vi "Get Next.vi"(0 "Stop Loop in":refnum<class "Stop Loop.lvclass">, 1 "Linked List Ref":refnum<data-value>, 5 "Active Unique ID":string, 9 "Active Element Index":i32, 11 "error in (no error)":errorcluster) -> (3 "Linked List Ref out":refnum<data-value>, 4 "Executioner out":refnum<class "Executioner.lvclass">, 6 "Active Unique ID out":string, 8 "Test Executive Ref out":refnum<data-value>, 10 "Active Element Index out":i32, 12 "Found":bool, 13 "Complete":bool, 14 "Stop":bool, 15 "error out":errorcluster)   [LabVIEW 2020, in "Test Executive.lvlib" / "Stop Loop.lvclass"]
uses:
  <vilib>/gpm_packages/@cs/test-executive/Source/Test Executive/Stop Loop/Stop Loop.lvclass
  C:/Program Files/National Instruments/LabVIEW 2020/vi.lib/gpm_packages/@cs/test-executive/Source/Test Executive/Executioner/Executioner.lvclass
  <vilib>/gpm_packages/@cs/test-executive/Source/Test Executive/Executioner/Executioner.lvclass
  <vilib>/gpm_packages/@cs/linked-list/Source/Linked List/ILinkedList/ILinked List.lvclass
  <vilib>/gpm_packages/@cs/test-executive/Source/Test Executive/ITestExecutive/ITest Executive.lvclass
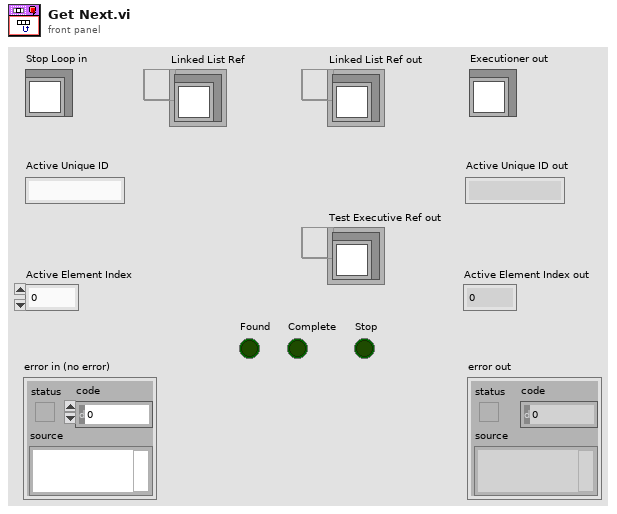
[diagram p1: front panel]
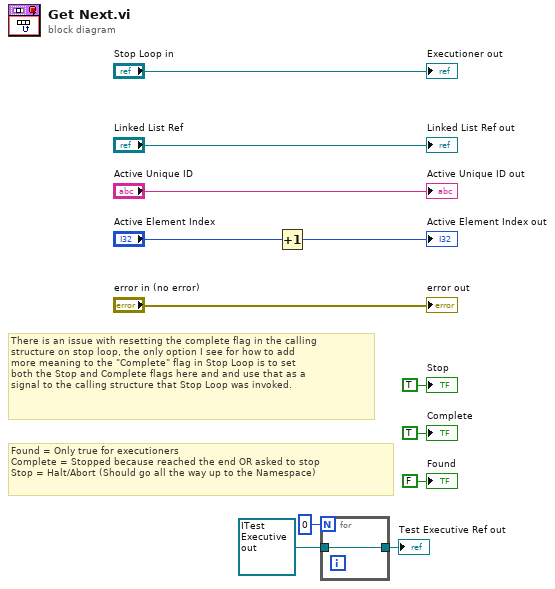
[diagram p0: block diagram]
diagram:
  # "There is an issue with resetting the complete flag in the calling\nstructure on stop loop, the only option I see for how to add\nmore meaning to the \"Complete\" flag in Stop Loop is to set\nboth the Stop and Complete flags here and and use that as a\nsignal to the calling structure that Stop Loop was invoked."
  # "Found = Only true for executioners\nComplete = Stopped because reached the end OR asked to stop\nStop = Halt/Abort (Should go all the way up to the Namespace)"
  n1 = Increment(x="Active Element Index") -> (x+1=→"Active Element Index out":i32)
  n2 = for {
    N: 0 -> [_]
    tunnel: refnum<data-value> refnum ("Test Executive Ref out") -> [w13]
    tunnel: [w13] -> w1
  }
  "Test Executive Ref out" <- w1
  "error out" <- "error in (no error)"
  "Executioner out" <- "Stop Loop in"
  "Linked List Ref out" <- "Linked List Ref"
  "Active Unique ID out" <- "Active Unique ID"
  "Found" <- FALSE ("Found")
  "Complete" <- TRUE ("Complete")
  "Stop" <- TRUE ("Stop")
